vi "运维调试_五参数.vi"() -> ()   [LabVIEW 2016, in "斯坦道仪器.lvlib"]
uses:
  <vilib>/Utility/miscctls.llb/LVPointTypeDef.ctl
  PLC/PLC.lvlib
panel:
  in  "打开串口":bool
  in  "释放串口":bool
  in  "手动通电":bool
  out "多参数横条运行状态":T1(xcontrol)
  in  "数据区":i32(listbox)
  in  "探头选择":u16(ring)=9 items=["氨氮"=3, "水温"=9, "pH值"=10, "溶解氧"=11, "电导率"=12, "浊度"=13, "叶绿素a"=14, "藻密度"=15, "蓝绿藻"=16, "氧化还原电位"=17, "溶解氧%"=18, "盐度"=19]
  in  "测量数据区读取":bool
  in  "测量数据区":i32(listbox)
  in  "状态告警区读取":bool
  in  "状态告警区":i32(listbox)
  in  "自动校准":bool
  in  "读取KB":bool
  in  "写入KB":bool
  out "B":dbl caption="校准值B:"
  out "K":dbl caption="校准值K:"
  in  "校准区探头选择":u16(ring)=9 items=["氨氮"=3, "水温"=9, "pH值"=10, "电导率"=12, "浊度"=13, "叶绿素a"=14, "藻密度"=15, "蓝绿藻"=16, "氧化还原电位"=17, "溶解氧%"=18, "盐度"=19]
  in  "停止测量(单探)":bool
  in  "启动测量(单探)":bool
  in  "控制命令区探头选择":u16(ring)=9 items=["氨氮"=3, "水温"=9, "pH值"=10, "溶解氧"=11, "电导率"=12, "浊度"=13, "叶绿素a"=14, "藻密度"=15, "蓝绿藻"=16, "氧化还原电位"=17, "溶解氧%"=18, "盐度"=19]
  in  "同步时间":bool
  in  "初始化(清洗)":bool
  in  "停止测量(全部)":bool
  in  "启动测量(全部)":bool
  in  "关键参数区读取":bool
  in  "关键参数区":i32(listbox)
  in  "传感器参数读取":bool
  in  "传感器区":i32(listbox)
  in  "返回":bool
  in  "设置":bool
  out "运行状态":string
  out "开机状态":bool
  in  "停止":bool
  in  "手动启动":bool
  out "集成报警信息":string
  # "控制命令区"
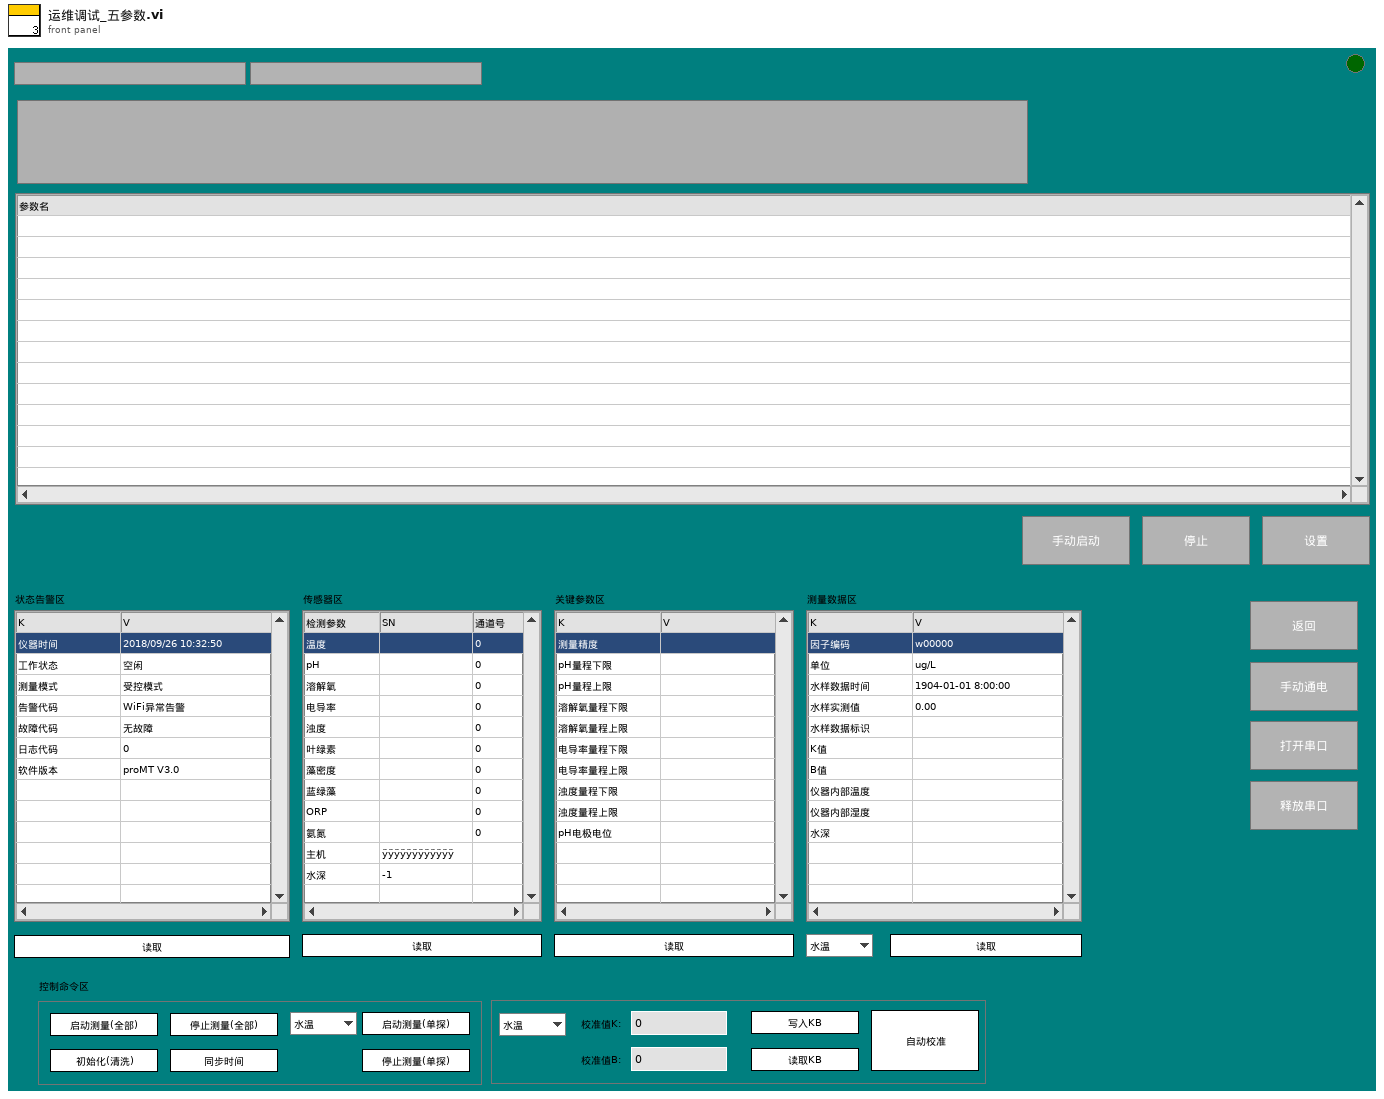
[diagram p1: front panel]
types:
  T1 = cluster{"系统时间":timestamp, "工作状态":u16, "测量模式":u16, "告警代码":enum16{"无告警", "缺试剂告警", "缺水样告警", "缺蒸馏水告警", "缺标液告警", "仪表漏液告警", "标定异常告警", "超量程告警", "加热异常", "低试剂预警", "超上限告警", "超下限告警", "仪表内部其他异常", "滴定异常告警", "电极异常告警", "量程切换告警", "参数设置告警", "PH电极电位异常", "电导率电极异常", "浊度光度异常", "溶解氧电极异常", "溶解氧光强异常", "温度异常告警", "PH异常告警", "溶解氧异常告警", "电导率异常告警", "浊度异常告警", "叶绿素异常告警", "藻密度异常告警", "蓝绿藻异常告警", "ORP异常告警", "氨氮异常告警", "清洁刷异常告警", "SD卡异常告警", "蓝牙异常告警", "Wifi异常告警", "流程异常告警"}, "故障代码":enum16{"无故障", "电机故障", "温度故障", "通讯故障", "滴定故障"}, "日志代码":u16, "软件版本":string}
  T2 = typedef "LVPointTypeDef.ctl" = cluster{"Horizontal":i16, "Vertical":i16}
  T3 = cluster{"时间标识":timestamp, "设备":string, "日志信息":string}
  T4 = enum16{"无告警", "缺试剂告警", "缺水样告警", "缺蒸馏水告警", "缺标液告警", "仪表漏液告警", "标定异常告警", "超量程告警", "加热异常", "低试剂预警", "超上限告警", "超下限告警", "仪表内部其他异常", "滴定异常告警", "电极异常告警", "量程切换告警", "参数设置告警", "PH电极电位异常", "电导率电极异常", "浊度光度异常", "溶解氧电极异常", "溶解氧光强异常", "温度异常告警", "PH异常告警", "溶解氧异常告警", "电导率异常告警", "浊度异常告警", "叶绿素异常告警", "藻密度异常告警", "蓝绿藻异常告警", "ORP异常告警", "氨氮异常告警", "清洁刷异常告警", "SD卡异常告警", "蓝牙异常告警", "Wifi异常告警", "流程异常告警"}
  T5 = cluster{"WORD[0]":u16, "WORD[1]":u16, "WORD[2]":u16, "WORD[3]":u16, "WORD[4]":u16, "WORD[5]":u16, "WORD[6]":u16, "WORD[7]":u16, "WORD[8]":u16, "WORD[9]":u16}
  T6 = cluster{"因子编码":string, "单位":string, "标样参考值":sgl, "水样数据时间":timestamp, "水样实测值":sgl, "水样数据标识":string, "K":sgl, "B":sgl, "T":sgl, "H":sgl, "水深":sgl}
  T7 = enum8{"Enabled", "Disabled", "Disabled and Grayed Out"}
  T8 = cluster{"测量模式":enum16{"待机", "水样测试", "标样核查", "零点核查", "跨度核查", "空白测试", "平行样测试", "加标回收", "空白校准", "标样校准", "初始化（清洗）"}, "数据标记表":string, "测量时间":dbl}
  T9 = cluster{"starting address":u16, "holding register value":u16}
  T10 = enum16{"idle", "init", "读状态", "读参数", "多个写入", "单个写入", "线圈写入"}
  T11 = enum32{"Bad", "Idle", "Run top level", "Running"}
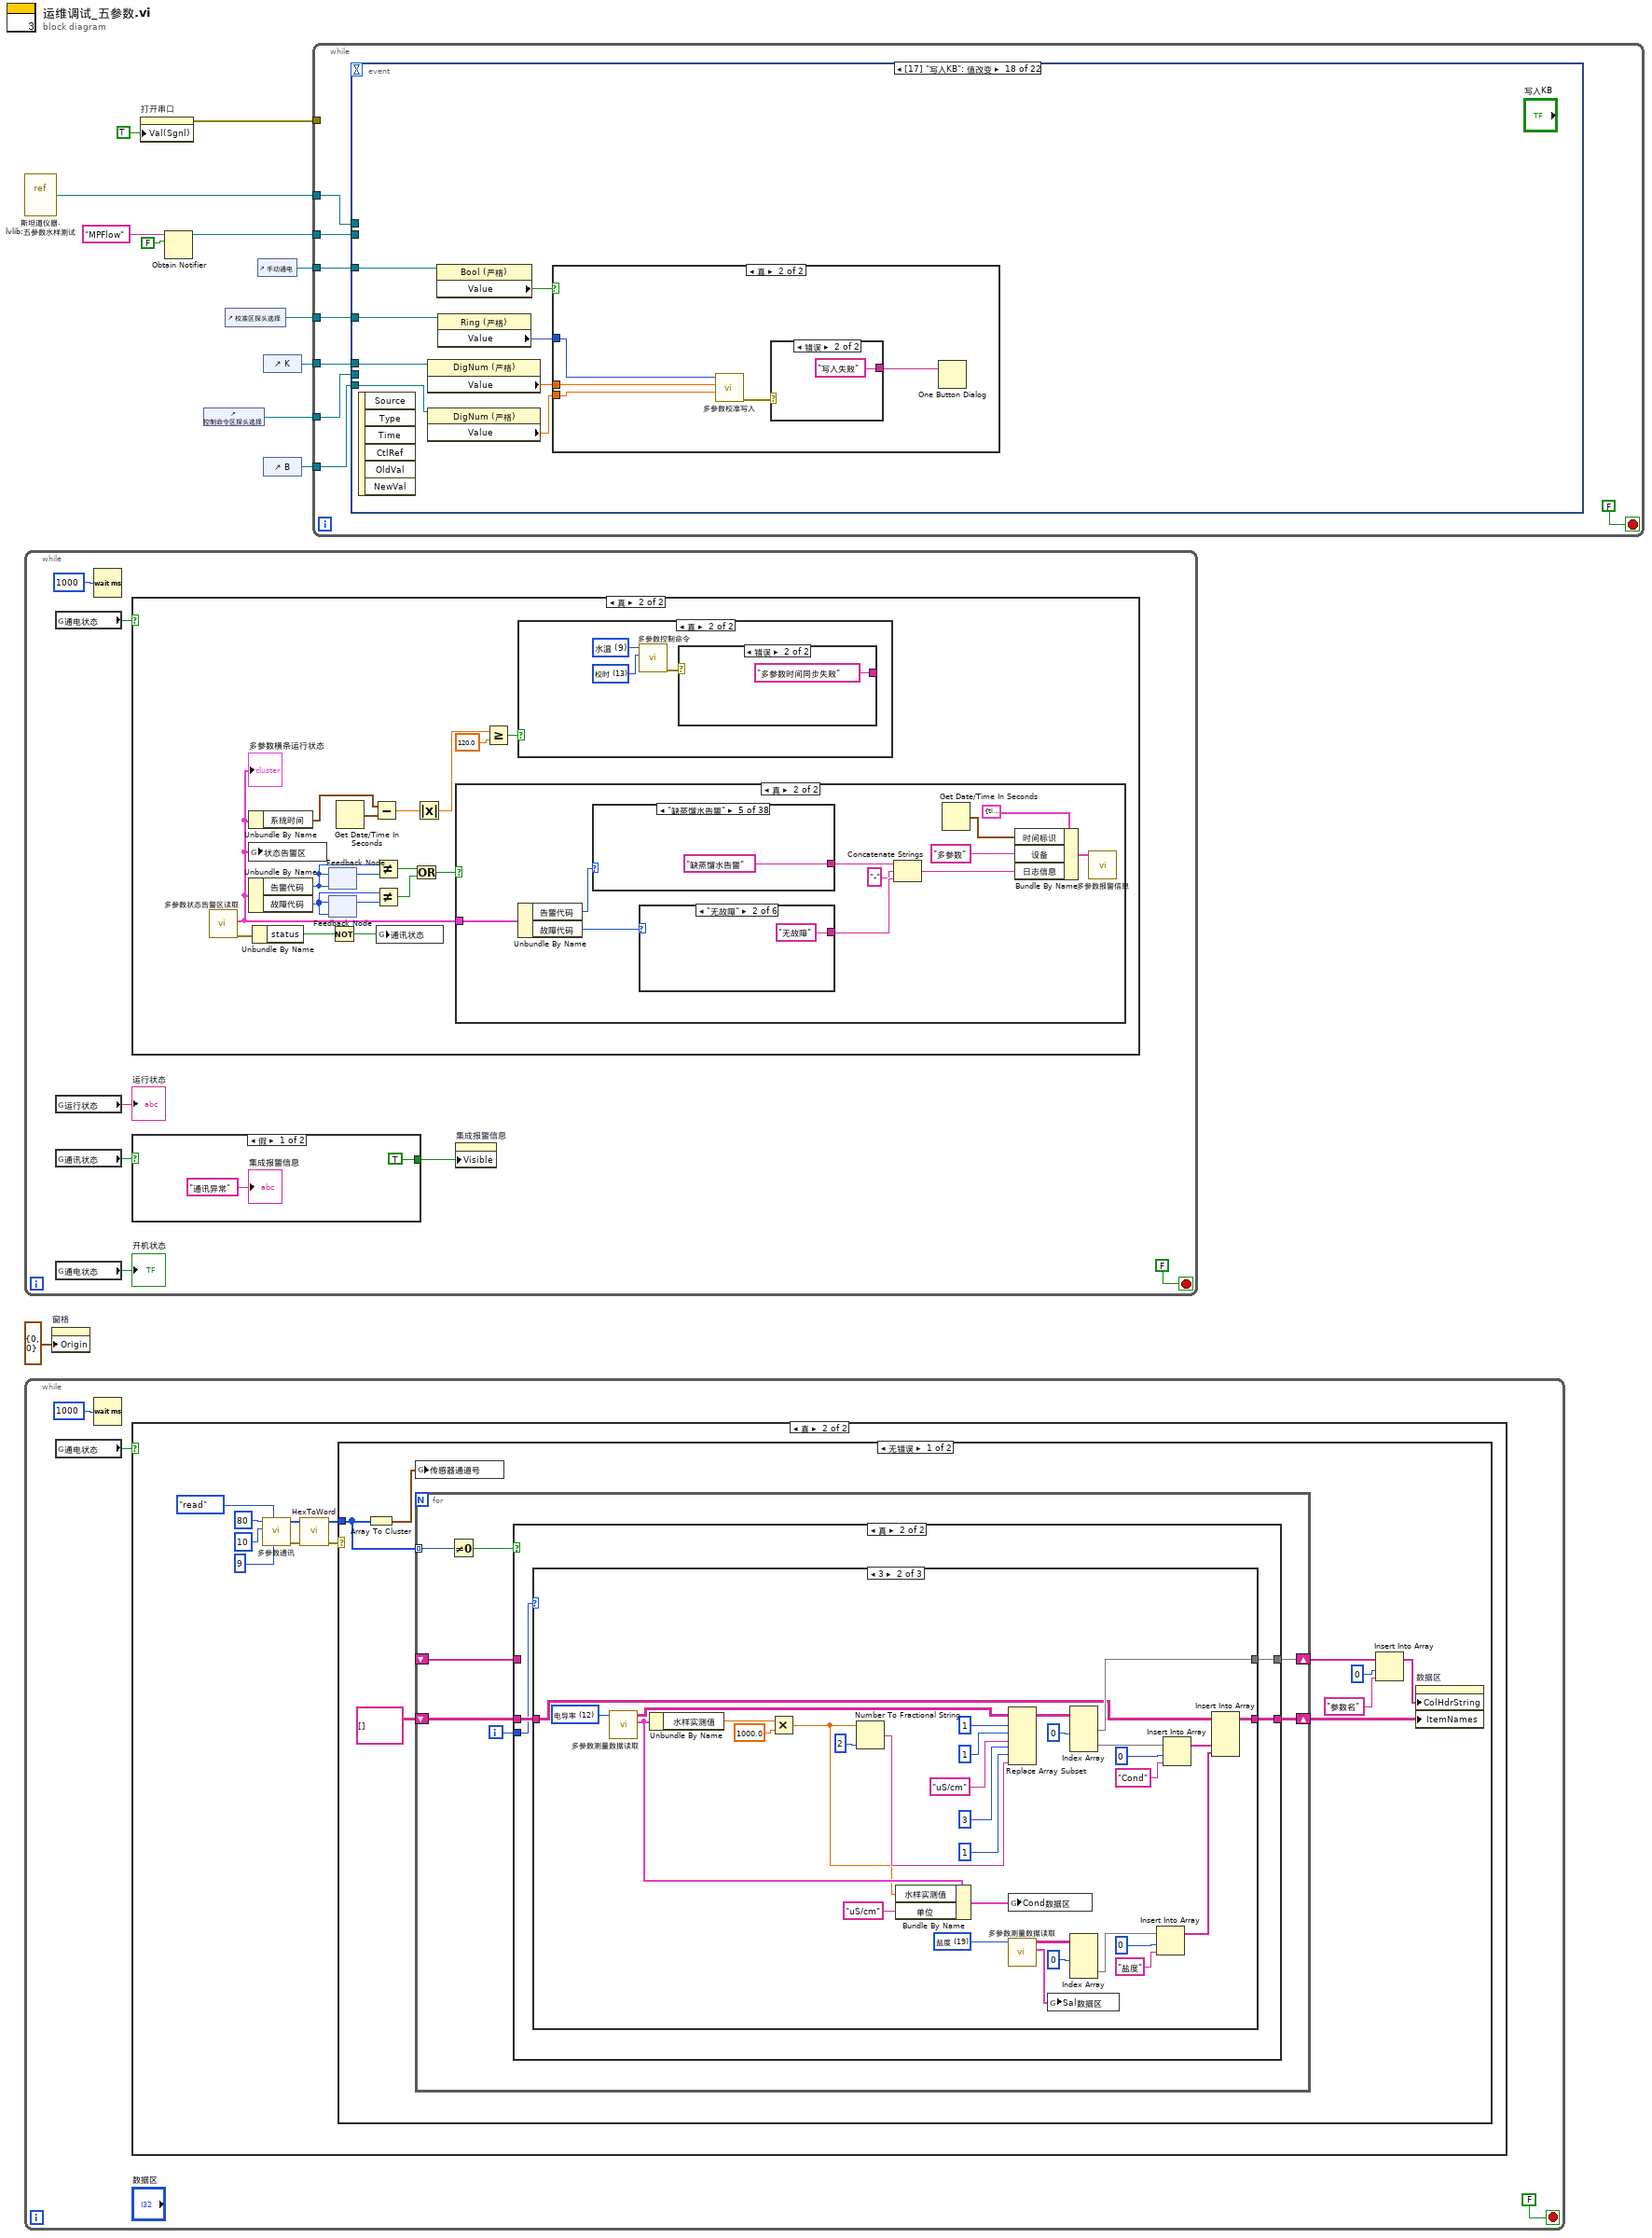
[diagram p0: block diagram]
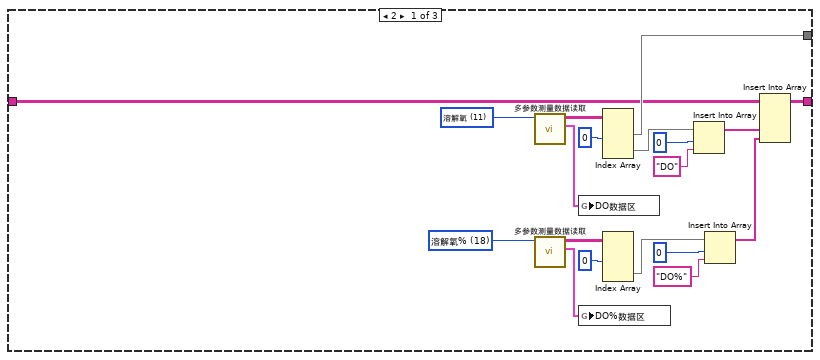
[diagram p4: hidden frame]
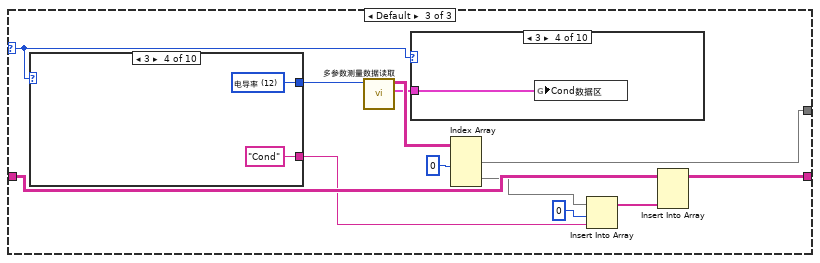
[diagram p5: hidden frame]
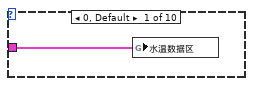
[diagram p6: hidden frame]
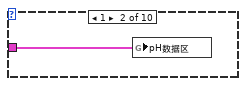
[diagram p7: hidden frame]
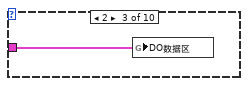
[diagram p8: hidden frame]
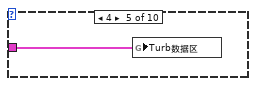
[diagram p9: hidden frame]
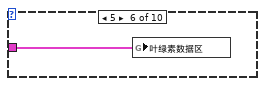
[diagram p10: hidden frame]
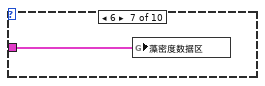
[diagram p11: hidden frame]
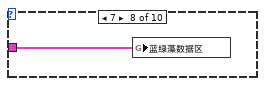
[diagram p12: hidden frame]
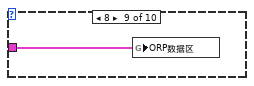
[diagram p13: hidden frame]
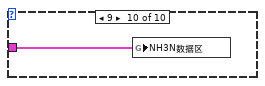
[diagram p14: hidden frame]
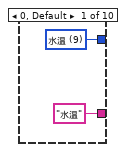
[diagram p15: hidden frame]
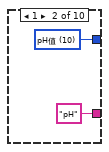
[diagram p16: hidden frame]
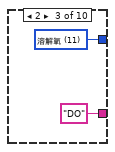
[diagram p17: hidden frame]
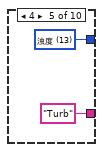
[diagram p18: hidden frame]
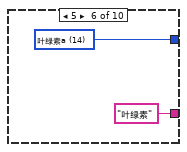
[diagram p19: hidden frame]
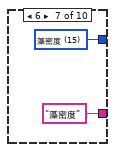
[diagram p20: hidden frame]
diagram:
  n1 = vi-ref "斯坦道仪器.lvlib:五参数水样测试.vi"() -> (w9:refnum<vi>)
  n2 = while {
    stop <- FALSE stop-if-true
    n3 = global read "多参数全局变量.vi" "通电状态"() -> (w13:bool)
    n4 = global read "多参数全局变量.vi" "运行状态"() -> (→"运行状态":string)
    n5 = global read "多参数全局变量.vi" "通讯状态"() -> (w17:bool)
    n6 = global read "多参数全局变量.vi" "通电状态"() -> (→"开机状态":bool)
    n7 = Wait (ms)(milliseconds to wait=u32 1000 ("等待时间（毫秒）")) -> ()  [unwired: 1 out]
    n8 = case shown="真" w13 {
      frame False {
      }
      frame True {
        n9 = call "多参数状态告警区读取.vi"() -> ("error out"=w29:errorcluster, "状态告警块"=w26:T1)  [unwired: 9 in, 1 out]
        "多参数横条运行状态" <- w26
        n10 = Unbundle By Name(w26) -> ("系统时间"=w25:timestamp)
        n11 = global write "多参数全局变量.vi" "状态告警区"(w26) -> ()
        n12 = Unbundle By Name(w26) -> ("告警代码"=w35:T4, "故障代码"=w33:enum16{"无故障", "电机故障", "温度故障", "通讯故障", "滴定故障"})
        n13 = Unbundle By Name(w29) -> ("status"=w28:bool)
        n14 = feedback #1(w35) -> (w36:T4)
        n15 = feedback-in #1(w35) -> ()
        n16 = feedback #2(w33) -> (w34:enum16{"无故障", "电机故障", "温度故障", "通讯故障", "滴定故障"})
        n17 = feedback-in #2(w33) -> ()
        n18 = Not(x=w28) -> (.not. x?=w27:bool)
        n19 = Get Date/Time In Seconds() -> (seconds since 1Jan1904=w24:timestamp)
        n20 = Subtract(x=w25, y=w24) -> (x-y=w23:dbl)
        n21 = Not Equal?(x=w35, y=w36) -> (x != y?=w31:bool)
        n22 = Not Equal?(x=w33, y=w34) -> (x != y?=w32:bool)
        n23 = global write "多参数全局变量.vi" "通讯状态"(w27) -> ()
        n24 = Or(x=w31, y=w32) -> (x .or. y?=w30:bool)
        n25 = Absolute Value(x=w23) -> (abs(x)=w22:dbl)
        n26 = case shown="真" w30 {
          tunnel: w26 -> [_ w52]
          frame False {
          }
          frame True {
            n27 = Unbundle By Name(w52) -> ("告警代码"=w51:T4, "故障代码"=w50:enum16{"无故障", "电机故障", "温度故障", "通讯故障", "滴定故障"})
            n28 = case shown="\"缺蒸馏水告警\"" w51 {
              selector: w51 -> [w63 _ _ _ _ _ _ _ _ _ _ _ _ _ _ _ _ _ _ _ _ _ _ _ _ _ _ _ _ _ _ _ _ _ _ _ _ _]
              tunnel: [w62 "无告警" "缺试剂告警" "缺水样告警" "缺蒸馏水告警" "缺标液告警" "仪表漏液告警" "标定异常告警" "超量程告警" "加热异常" "低试剂预警" "超上限告警" "超下限告警" "仪表内部其他异常" "滴定异常告警" "电极异常告警" "量程切换告警" "参数设置告警" "PH电极电位异常" "电导率电极异常" "浊度光度异常" "溶解氧电极异常" "溶解氧光强异常" "温度异常告警" "PH异常告警" "溶解氧异常告警" "电导率异常告警" "浊度异常告警" "叶绿素异常告警" "藻密度异常告警" "蓝绿藻异常告警" "ORP异常告警" "氨氮异常告警" "清洁刷异常告警" "SD卡异常告警" "蓝牙异常告警" "WiFi异常告警" "流程异常告警"] -> w49
              frame Default {
                n29 = Format Into String(format string="%d" ("格式字符串"), initial string="未知" ("工作状态"), w63) -> (resulting string=w62:string)  [unwired: 1 in, 1 out]
              }
              frame "无告警" {
              }
              frame "缺试剂告警" {
              }
              frame "缺水样告警" {
              }
              frame "缺蒸馏水告警" {
              }
              frame "缺标液告警" {
              }
              frame "仪表漏液告警" {
              }
              frame "标定异常告警" {
              }
              frame "超量程告警" {
              }
              frame "加热异常" {
              }
              frame "低试剂预警" {
              }
              frame "超上限告警" {
              }
              frame "超下限告警" {
              }
              frame "仪表内部其他异常" {
              }
              frame "滴定异常告警" {
              }
              frame "电极异常告警" {
              }
              frame "量程切换告警" {
              }
              frame "参数设置告警" {
              }
              frame "PH电极电位异常" {
              }
              frame "电导率电极异常" {
              }
              frame "浊度光度异常" {
              }
              frame "溶解氧电极异常" {
              }
              frame "溶解氧光强异常" {
              }
              frame "温度异常告警" {
              }
              frame "PH异常告警" {
              }
              frame "溶解氧异常告警" {
              }
              frame "电导率异常告警" {
              }
              frame "浊度异常告警" {
              }
              frame "叶绿素异常告警" {
              }
              frame "藻密度异常告警" {
              }
              frame "蓝绿藻异常告警" {
              }
              frame "ORP异常告警" {
              }
              frame "氨氮异常告警" {
              }
              frame "清洁刷异常告警" {
              }
              frame "SD卡异常告警" {
              }
              frame "蓝牙异常告警" {
              }
              frame "Wifi异常告警" {
              }
              frame "流程异常告警" {
              }
            }
            n30 = case shown="\"无故障\"" w50 {
              selector: w50 -> [w54 _ _ _ _ _]
              tunnel: [w53 "无故障" "电机故障" "温度故障" "通讯故障" "滴定故障"] -> w48
              frame Default {
                n31 = Format Into String(format string="%d" ("格式字符串"), initial string="未知" ("工作状态"), w54) -> (resulting string=w53:string)  [unwired: 1 in, 1 out]
              }
              frame "无故障" {
              }
              frame "电机故障" {
              }
              frame "温度故障" {
              }
              frame "通讯故障" {
              }
              frame "滴定故障" {
              }
            }
            n32 = Concatenate Strings(w49, "-" ("字符串"), w48) -> (w44:string)
            n33 = Get Date/Time In Seconds() -> (seconds since 1Jan1904=w43:timestamp)
            n34 = Bundle By Name(cluster=T3 {"时间标识"=timestamp(0 s since 1904-01-01), "设备"="", "日志信息"=""} ("data in"), "时间标识"=w43, "设备"="多参数", "日志信息"=w44) -> (w45:T3)
            n35 = call "多参数报警信息.vi"("data in"=w45) -> ()  [unwired: 10 in, 1 out]
          }
        }
        n36 = Greater Or Equal?(x=w22, y=120.0) -> (x >= y?=w21:bool)
        n37 = case shown="真" w21 {
          frame False {
          }
          frame True {
            w37 = u16 13 items=["启动测量（全部）"=1, "初始化（清洗）"=10, "停止测量（全部）"=11, "校时"=13, "启动测量（单个传感器）"=19, "停止测量（单个传感器）"=20] ("控制命令")
            w38 = u16 9 items=["氨氮"=3, "水温"=9, "pH值"=10, "溶解氧"=11, "电导率"=12, "浊度"=13, "叶绿素a"=14, "藻密度"=15, "蓝绿藻"=16, "氧化还原电位"=17, "溶解氧%"=18, "盐度"=19] ("站号")
            n38 = call "多参数控制命令.vi"("控制命令"=w37, "站号"=w38) -> ("error out"=w39:errorcluster)  [unwired: 9 in]
            n39 = case shown="错误" w39 {
              tunnel: ["多参数时间同步成功" ("消息") "多参数时间同步失败" ("消息")] -> _
              frame No Error {
              }
              frame Error {
              }
            }
          }
        }
      }
    }
    n40 = case shown="假" w17 {
      tunnel: [TRUE ("可见") _] -> w16
      frame False {
        "集成报警信息" <- "通讯异常" ("集成报警信息")
      }
      frame True {
      }
    }
    n41 = property on="集成报警信息" class="Str"("Visible"=w16) -> ()  [unwired: 2 in, 2 out]
  }
  n42 = while {
    stop <- FALSE stop-if-true
    n43 = global read "多参数全局变量.vi" "通电状态"() -> (w105:bool)
    n44 = Wait (ms)(milliseconds to wait=u32 1000 ("等待时间（毫秒）")) -> ()  [unwired: 1 out]
    n45 = case shown="真" w105 {
      frame False {
      }
      frame True {
        n46 = call "多参数通讯.vi"("Slave ID"=u8 9, "STEP"=enum16{"open", "read", "write", "close"}."read", "quantity"=u16 10, "starting address"=u16 80) -> ("error out"=w110:errorcluster, "Registers"=w111:u16[])  [unwired: 5 in, 1 out]
        n47 = call "HexToWord.vi"("数组"=w111) -> ("WORD"=w114:u16[])  [unwired: 10 in]
        n48 = case shown="无错误" w110 {
          tunnel: w114 -> [w115 _]
          frame No Error {
            n49 = Array To Cluster(array=w115) -> (cluster=w116:T5)
            n50 = global write "多参数全局变量.vi" "传感器通道号"(w116) -> ()
            n51 = for {
              tunnel: w115 -> [w128] mode=indexing
              shift-right: [w126] -> w120
              shift-left: _ -> [w125]
              shift-right: [w123] -> w121
              shift-left: string[][] [] ("子数组") -> [w124]
              i -> [w129]
              n52 = Not Equal To 0?(x=w128) -> (x != 0?=w127:bool)
              n53 = case shown="真" w127 {
                tunnel: w129 -> [_ w132]
                tunnel: [w131 w135] -> w126
                tunnel: w125 -> [w131 _]
                tunnel: w124 -> [w130 w134]
                tunnel: [w130 w133] -> w123
                frame False {
                }
                frame True {
                  n54 = case shown="3" w132 {
                    selector: w132 -> [_ _ w187]
                    tunnel: [w144 w176 w195] -> w135
                    tunnel: w134 -> [w140 w174 w194]
                    tunnel: [w143 w162 w193] -> w133
                    frame 2 {
                      w138 = u16 18 items=["氨氮"=3, "水温"=9, "pH值"=10, "溶解氧"=11, "电导率"=12, "浊度"=13, "叶绿素a"=14, "藻密度"=15, "蓝绿藻"=16, "氧化还原电位"=17, "溶解氧%"=18, "盐度"=19] ("探头选择")
                      w139 = u16 11 items=["氨氮"=3, "水温"=9, "pH值"=10, "溶解氧"=11, "电导率"=12, "浊度"=13, "叶绿素a"=14, "藻密度"=15, "蓝绿藻"=16, "氧化还原电位"=17, "溶解氧%"=18, "盐度"=19] ("探头选择")
                      n55 = call "多参数测量数据读取.vi"("探头选择"=w139) -> ("测量数据块"=w137:T6, "添加的数组"=w142:string[][])  [unwired: 8 in, 1 out]
                      n56 = call "多参数测量数据读取.vi"("探头选择"=w138) -> ("测量数据块"=w136:T6, "添加的数组"=w141:string[][])  [unwired: 8 in, 1 out]
                      n57 = global write "多参数全局变量.vi" "DO数据区"(w137) -> ()
                      n58 = global write "多参数全局变量.vi" "DO%数据区"(w136) -> ()
                      n59 = Index Array(array=w142, index (col) #1=0 ("禁用的索引 (列)")) -> (element #1=w144:string[], element #2=w153:string[])  [unwired: 3 in]
                      n60 = Index Array(array=w141, index (col) #1=0 ("禁用的索引 (列)")) -> (element #2=w149:string[])  [unwired: 3 in, 1 out]
                      n61 = Insert Into Array(array=w153, index=0 ("索引"), new element="DO") -> (w151:string[])
                      n62 = Insert Into Array(array=w149, index=0 ("索引"), new element="DO%") -> (w148:string[])
                      n63 = Insert Into Array(array=w140, new element #1=w151, new element #2=w148) -> (w143:string[][])  [unwired: 2 in]
                    }
                    frame 3 {
                      w172 = u16 19 items=["氨氮"=3, "水温"=9, "pH值"=10, "溶解氧"=11, "电导率"=12, "浊度"=13, "叶绿素a"=14, "藻密度"=15, "蓝绿藻"=16, "氧化还原电位"=17, "溶解氧%"=18, "盐度"=19] ("探头选择")
                      w173 = u16 12 items=["氨氮"=3, "水温"=9, "pH值"=10, "溶解氧"=11, "电导率"=12, "浊度"=13, "叶绿素a"=14, "藻密度"=15, "蓝绿藻"=16, "氧化还原电位"=17, "溶解氧%"=18, "盐度"=19] ("探头选择")
                      n64 = call "多参数测量数据读取.vi"("探头选择"=w173) -> ("测量数据块"=w168:T6, "添加的数组"=w160:string[][])  [unwired: 8 in, 1 out]
                      n65 = Unbundle By Name(w168) -> ("水样实测值"=w170:sgl)
                      n66 = Multiply(x=w170, y=sgl 1000.0) -> (x*y=w155:sgl)
                      n67 = Number To Fractional String(number=w155, precision (6)=i16 2 ("精度(6)")) -> (F-format string=w156:string)  [unwired: 2 in]
                      n68 = Bundle By Name(cluster=w168, "水样实测值"=w155, "单位"="uS/cm") -> (w166:T6)
                      n69 = Replace Array Subset(array=w160, new element #1="uS/cm" ("新元素/子数组"), index (row) #1=1 ("索引 (行)"), index (col) #1=1 ("禁用的索引 (列)"), new element #2=w156, index (row) #2=3 ("索引 (行)"), index (col) #2=1 ("禁用的索引 (列)")) -> (w161:string[][])
                      n70 = global write "多参数全局变量.vi" "Cond数据区"(w166) -> ()
                      n71 = call "多参数测量数据读取.vi"("探头选择"=w172) -> ("测量数据块"=w171:T6, "添加的数组"=w175:string[][])  [unwired: 8 in, 1 out]
                      n72 = global write "多参数全局变量.vi" "Sal数据区"(w171) -> ()
                      n73 = Index Array(array=w161, index (col) #1=0 ("禁用的索引 (列)")) -> (element #1=w176:string[], element #2=w185:string[])  [unwired: 3 in]
                      n74 = Index Array(array=w175, index (col) #1=0 ("禁用的索引 (列)")) -> (element #2=w181:string[])  [unwired: 3 in, 1 out]
                      n75 = Insert Into Array(array=w181, index=0 ("索引"), new element="盐度") -> (w180:string[])
                      n76 = Insert Into Array(array=w185, index=0 ("索引"), new element="Cond") -> (w183:string[])
                      n77 = Insert Into Array(array=w174, new element #1=w183, new element #2=w180) -> (w162:string[][])  [unwired: 2 in]
                    }
                    frame Default {
                      n78 = case shown="3" w187 {
                        tunnel: [w210 w212 w214 w216 w218 w220 w222 w224 w226 w228] -> w198
                        tunnel: ["水温" "pH" "DO" "Cond" "Turb" "叶绿素" "藻密度" "蓝绿藻" "ORP" "氨氮"] -> w191
                        frame 0, Default {
                          w210 = u16 9 items=["氨氮"=3, "水温"=9, "pH值"=10, "溶解氧"=11, "电导率"=12, "浊度"=13, "叶绿素a"=14, "藻密度"=15, "蓝绿藻"=16, "氧化还原电位"=17, "溶解氧%"=18, "盐度"=19] ("探头选择")
                        }
                        frame 1 {
                          w212 = u16 10 items=["氨氮"=3, "水温"=9, "pH值"=10, "溶解氧"=11, "电导率"=12, "浊度"=13, "叶绿素a"=14, "藻密度"=15, "蓝绿藻"=16, "氧化还原电位"=17, "溶解氧%"=18, "盐度"=19] ("探头选择")
                        }
                        frame 2 {
                          w214 = u16 11 items=["氨氮"=3, "水温"=9, "pH值"=10, "溶解氧"=11, "电导率"=12, "浊度"=13, "叶绿素a"=14, "藻密度"=15, "蓝绿藻"=16, "氧化还原电位"=17, "溶解氧%"=18, "盐度"=19] ("探头选择")
                        }
                        frame 3 {
                          w216 = u16 12 items=["氨氮"=3, "水温"=9, "pH值"=10, "溶解氧"=11, "电导率"=12, "浊度"=13, "叶绿素a"=14, "藻密度"=15, "蓝绿藻"=16, "氧化还原电位"=17, "溶解氧%"=18, "盐度"=19] ("探头选择")
                        }
                        frame 4 {
                          w218 = u16 13 items=["氨氮"=3, "水温"=9, "pH值"=10, "溶解氧"=11, "电导率"=12, "浊度"=13, "叶绿素a"=14, "藻密度"=15, "蓝绿藻"=16, "氧化还原电位"=17, "溶解氧%"=18, "盐度"=19] ("探头选择")
                        }
                        frame 5 {
                          w220 = u16 14 items=["氨氮"=3, "水温"=9, "pH值"=10, "溶解氧"=11, "电导率"=12, "浊度"=13, "叶绿素a"=14, "藻密度"=15, "蓝绿藻"=16, "氧化还原电位"=17, "溶解氧%"=18, "盐度"=19] ("探头选择")
                        }
                        frame 6 {
                          w222 = u16 15 items=["氨氮"=3, "水温"=9, "pH值"=10, "溶解氧"=11, "电导率"=12, "浊度"=13, "叶绿素a"=14, "藻密度"=15, "蓝绿藻"=16, "氧化还原电位"=17, "溶解氧%"=18, "盐度"=19] ("探头选择")
                        }
                        frame 7 {
                          w224 = u16 16 items=["氨氮"=3, "水温"=9, "pH值"=10, "溶解氧"=11, "电导率"=12, "浊度"=13, "叶绿素a"=14, "藻密度"=15, "蓝绿藻"=16, "氧化还原电位"=17, "溶解氧%"=18, "盐度"=19] ("探头选择")
                        }
                        frame 8 {
                          w226 = u16 17 items=["氨氮"=3, "水温"=9, "pH值"=10, "溶解氧"=11, "电导率"=12, "浊度"=13, "叶绿素a"=14, "藻密度"=15, "蓝绿藻"=16, "氧化还原电位"=17, "溶解氧%"=18, "盐度"=19] ("探头选择")
                        }
                        frame 9 {
                          w228 = u16 3 items=["氨氮"=3, "水温"=9, "pH值"=10, "溶解氧"=11, "电导率"=12, "浊度"=13, "叶绿素a"=14, "藻密度"=15, "蓝绿藻"=16, "氧化还原电位"=17, "溶解氧%"=18, "盐度"=19] ("探头选择")
                        }
                      }
                      n79 = call "多参数测量数据读取.vi"("探头选择"=w198) -> ("测量数据块"=w188:T6, "添加的数组"=w197:string[][])  [unwired: 8 in, 1 out]
                      n80 = case shown="3" w187 {
                        tunnel: w188 -> [w199 w200 w201 w202 w203 w204 w205 w206 w207 w208]
                        frame 0, Default {
                          n81 = global write "多参数全局变量.vi" "水温数据区"(w199) -> ()
                        }
                        frame 1 {
                          n82 = global write "多参数全局变量.vi" "pH数据区"(w200) -> ()
                        }
                        frame 2 {
                          n83 = global write "多参数全局变量.vi" "DO数据区"(w201) -> ()
                        }
                        frame 3 {
                          n84 = global write "多参数全局变量.vi" "Cond数据区"(w202) -> ()
                        }
                        frame 4 {
                          n85 = global write "多参数全局变量.vi" "Turb数据区"(w203) -> ()
                        }
                        frame 5 {
                          n86 = global write "多参数全局变量.vi" "叶绿素数据区"(w204) -> ()
                        }
                        frame 6 {
                          n87 = global write "多参数全局变量.vi" "藻密度数据区"(w205) -> ()
                        }
                        frame 7 {
                          n88 = global write "多参数全局变量.vi" "蓝绿藻数据区"(w206) -> ()
                        }
                        frame 8 {
                          n89 = global write "多参数全局变量.vi" "ORP数据区"(w207) -> ()
                        }
                        frame 9 {
                          n90 = global write "多参数全局变量.vi" "NH3N数据区"(w208) -> ()
                        }
                      }
                      n91 = Index Array(array=w197, index (col) #1=0 ("禁用的索引 (列)")) -> (element #1=w195:string[], element #2=w192:string[])  [unwired: 3 in]
                      n92 = Insert Into Array(array=w192, index=0 ("索引"), new element=w191) -> (w190:string[])
                      n93 = Insert Into Array(array=w194, new element=w190) -> (w193:string[][])  [unwired: 2 in]
                    }
                  }
                }
              }
            }
            n94 = Insert Into Array(array=w120, index=0 ("索引"), new element="参数名" ("新元素/子数组")) -> (w119:string[])
            n95 = property on="数据区" class="MCListbox (严格)"("ColHdrString"=w119, "ItemNames"=w121) -> ()  [unwired: 2 in, 2 out]
          }
          frame Error {
          }
        }
      }
    }
  }
  n96 = property on="窗格" class="Pane"("Origin"=T2 {"Horizontal"=0, "Vertical"=0} ("原点")) -> ()  [unwired: 2 in, 2 out]
  n97 = property on="打开串口" class="Bool (严格)"("Val(Sgnl)"=TRUE ("值(信号)")) -> (error out=w1:errorcluster)  [unwired: 2 in, 1 out]
  n98 = Obtain Notifier(name (unnamed)="MPFlow" ("名称（未命名）"), notification data type=FALSE) -> (notifier out=w8:refnum<notifier>)  [unwired: 2 in, 2 out]
  n99 = control-ref of="控制命令区探头选择"() -> (w7:refnum<vi>)
  n100 = control-ref of="校准区探头选择"() -> (w4:refnum<vi>)
  n101 = control-ref of="手动通电"() -> (w3:refnum<vi>)
  n102 = control-ref of="K"() -> (w6:refnum<vi>)
  n103 = control-ref of="B"() -> (w5:refnum<vi>)
  n104 = while {
    tunnel: w9 -> [w235]
    tunnel: w8 -> [w234]
    tunnel: w7 -> [w233]
    tunnel: w6 -> [w232]
    tunnel: w5 -> [w231]
    tunnel: w4 -> [w230]
    tunnel: w3 -> [w229]
    tunnel: w1 -> [_]
    stop <- FALSE stop-if-true
    n105 = event shown="[17] \"写入KB\": 值改变" {
      selector: _ -> [_ _ _ _ _ _ _ _ _ _ _ _ _ _ _ _ _ _ _ _ _ _]
      dyn-events: _ -> [_ _ _ _ _ _ _ _ _ _ _ _ _ _ _ _ _ _ _ _ _ _]
      timeout: _ -> [_ _ _ _ _ _ _ _ _ _ _ _ _ _ _ _ _ _ _ _ _ _]
      tunnel: w235 -> [_ _ _ w251 _ _ _ _ _ _ _ _ _ _ _ _ _ _ _ _ _ _]
      tunnel: w234 -> [_ _ _ _ w273 _ _ _ _ _ _ _ _ _ _ _ _ _ _ _ _ _]
      tunnel: w233 -> [_ _ _ _ _ _ _ _ _ _ _ _ _ _ _ w337 w351 _ _ _ _ _]
      tunnel: w232 -> [_ _ _ _ _ _ _ _ _ _ _ _ _ _ _ _ _ w362 _ _ _ _]
      tunnel: w231 -> [_ _ _ _ _ _ _ _ _ _ _ _ _ _ _ _ _ w364 _ _ _ _]
      tunnel: w230 -> [_ _ _ _ _ _ _ _ _ _ _ _ _ _ _ _ _ w366 _ w382 _ _]
      tunnel: w229 -> [_ _ _ _ _ _ _ w281 w286 w291 w297 w302 w311 w320 w329 w339 w349 w360 _ w380 w392 _]
      event Timeout {
        n106 = event-data() -> ()  [unwired: 1 in, 3 out]
      }
      event "释放串口": Value Change {
        n107 = event-data() -> ("NewVal"=w237:bool)  [unwired: 1 in, 5 out]
        n108 = case shown="真" w237 {
          frame False {
          }
          frame True {
            n109 = call "多参数通讯.vi"("STEP"=enum16{"open", "read", "write", "close"}."close") -> ("error out"=w238:errorcluster)  [unwired: 8 in, 2 out]
            n110 = case shown="无错误" w238 {
              frame No Error {
                n111 = property on="打开串口" class="Bool (严格)"("DisabledEnum"=T7."Enabled" ("禁用")) -> ()  [unwired: 2 in, 2 out]
              }
              frame Error {
              }
            }
          }
        }
      }
      event "打开串口": Value Change {
        n112 = event-data() -> ("NewVal"=w241:bool)  [unwired: 1 in, 5 out]
        n113 = case shown="真" w241 {
          frame False {
          }
          frame True {
            n114 = call "多参数通讯.vi"("STEP"=enum16{"open", "read", "write", "close"}."open") -> ("error out"=w242:errorcluster)  [unwired: 8 in, 2 out]
            n115 = case shown="错误" w242 {
              tunnel: [T7."Disabled and Grayed Out" ("禁用") T7."Enabled" ("禁用")] -> w244
              frame No Error {
              }
              frame Error {
                n116 = One Button Dialog(message="多参数串口打开失败" ("消息")) -> ()  [unwired: 1 in, 1 out]
              }
            }
            n117 = property on="打开串口" class="Bool (严格)"("DisabledEnum"=w244, "Value"=FALSE ("打开串口")) -> ()  [unwired: 2 in, 2 out]
          }
        }
      }
      event "手动启动": Value Change {
        n118 = event-data() -> ()  [unwired: 1 in, 6 out]
        n119 = call "多参数启动参数对话框.vi"() -> ("确认"=w250:bool, "测量时间"=w249:dbl)  [unwired: 10 in]
        n120 = case shown="真" w250 {
          tunnel: w251 -> [_ w253]
          tunnel: w249 -> [_ w252]
          frame False {
          }
          frame True {
            n121 = property class="VI"(reference=w253) -> ("Name"=w257:string, "Exec.State"=w255:T11)  [unwired: 1 in, 2 out]
            n122 = Open VI Reference(type specifier VI Refnum (for type only)=refnum<vi> refnum ("类型说明符VI引用句柄（仅用于类型）"), vi path=w257, options=128 ("选项")) -> (vi reference=w256:refnum<vi>)  [unwired: 3 in, 1 out]
            n123 = case shown="\"Idle\"" w255 {
              tunnel: w256 -> [w261 w268]
              tunnel: [w261 w267] -> w254
              tunnel: w252 -> [_ w262]
              frame "Bad", Default {
                n124 = One Button Dialog(message="仪器已经启动，无需重复启动" ("消息")) -> ()  [unwired: 1 in, 1 out]
              }
              frame "Idle" {
                n125 = global read "系统变量.vi" "运行模式"() -> (w264:enum16{"维护模式", "常规模式", "应急模式", "质控模式"})
                n126 = case shown="\"常规模式\", 默认" w264 {
                  tunnel: ["M" ("数据标记表") "hd" ("数据标记表")] -> w263
                  frame "维护模式" {
                  }
                  frame "常规模式", Default {
                  }
                }
                n127 = Bundle By Name(cluster=T8 {"测量模式"=enum."水样测试", "数据标记表"="", "测量时间"=0.0} ("启动参数"), "数据标记表"=w263, "测量时间"=w262) -> (w265:T8)
                n128 = call-by-ref "开始异步调用"(reference=w268, "启动参数"=w265) -> (reference out=w267:refnum<vi>)  [unwired: 12 in, 1 out]
              }
            }
            n129 = Close Reference(reference=w254) -> ()  [unwired: 1 in, 1 out]
          }
        }
      }
      event "停止": Value Change {
        n130 = event-data() -> ()  [unwired: 1 in, 6 out]
        n131 = Two Button Dialog(message="请再一次确认是否停止测量" ("消息")) -> (T button?=w271:bool)  [unwired: 2 in]
        n132 = case shown="真" w271 {
          tunnel: w273 -> [_ w276]
          frame False {
          }
          frame True {
            w274 = u16 11 items=["启动测量（全部）"=1, "初始化（清洗）"=10, "停止测量（全部）"=11, "校时"=13, "启动测量（单个传感器）"=19, "停止测量（单个传感器）"=20] ("控制命令")
            w275 = u16 10 items=["氨氮"=3, "水温"=9, "pH值"=10, "溶解氧"=11, "电导率"=12, "浊度"=13, "叶绿素a"=14, "藻密度"=15, "蓝绿藻"=16, "氧化还原电位"=17, "溶解氧%"=18, "盐度"=19] ("站号")
            n133 = Send Notification(notification=TRUE ("通知"), notifier=w276) -> ()  [unwired: 1 in, 2 out]
            n134 = call "多参数控制命令.vi"("控制命令"=w274, "站号"=w275) -> ()  [unwired: 9 in, 1 out]
          }
        }
      }
      event "设置": Value Change {
        n135 = event-data() -> ()  [unwired: 1 in, 6 out]
        n136 = property on="窗格" class="Pane"("Origin"=T2 {"Horizontal"=0, "Vertical"=528} ("原点")) -> ()  [unwired: 2 in, 2 out]
      }
      event "返回": Value Change {
        n137 = event-data() -> ()  [unwired: 1 in, 6 out]
        n138 = property on="窗格" class="Pane"("Origin"=T2 {"Horizontal"=0, "Vertical"=0} ("原点")) -> ()  [unwired: 2 in, 2 out]
      }
      event "传感器参数读取": Value Change {
        n139 = event-data() -> ()  [unwired: 1 in, 6 out]
        n140 = property class="Bool (严格)"(reference=w281) -> ("Value"=w280:bool)  [unwired: 1 in, 2 out]
        n141 = case shown="真" w280 {
          frame False {
            n142 = One Button Dialog(message="启动失败，请先通电" ("消息")) -> ()  [unwired: 1 in, 1 out]
          }
          frame True {
            n143 = call "多参数传感器参数读取.vi"() -> ("error out"=w283:errorcluster, "添加的数组"=w284:string[][])  [unwired: 10 in]
            n144 = call <vilib>:"General Error Handler.vi"("error in (no error)"=w283) -> ()  [unwired: 10 in, 5 out]
            n145 = property on="传感器区" class="MCListbox (严格)"("ItemNames"=w284) -> ()  [unwired: 2 in, 2 out]
          }
        }
      }
      event "关键参数区读取": Value Change {
        n146 = event-data() -> ()  [unwired: 1 in, 6 out]
        n147 = property class="Bool (严格)"(reference=w286) -> ("Value"=w285:bool)  [unwired: 1 in, 2 out]
        n148 = case shown="假" w285 {
          frame False {
            n149 = One Button Dialog(message="启动失败，请先通电" ("消息")) -> ()  [unwired: 1 in, 1 out]
          }
          frame True {
            n150 = call "多参数关键参数读取.vi"() -> ("error out"=w288:errorcluster, "添加的数组"=w289:string[][])  [unwired: 10 in]
            n151 = call <vilib>:"General Error Handler.vi"("error in (no error)"=w288) -> ()  [unwired: 10 in, 5 out]
            n152 = property on="关键参数区" class="MCListbox (严格)"("ItemNames"=w289) -> ()  [unwired: 2 in, 2 out]
          }
        }
      }
      event "测量数据区读取": Value Change {
        n153 = event-data() -> ()  [unwired: 1 in, 6 out]
        n154 = property class="Bool (严格)"(reference=w291) -> ("Value"=w290:bool)  [unwired: 1 in, 2 out]
        n155 = case shown="假" w290 {
          frame False {
            n156 = One Button Dialog(message="启动失败，请先通电" ("消息")) -> ()  [unwired: 1 in, 1 out]
          }
          frame True {
            n157 = call "多参数测量数据读取.vi"("探头选择"="探头选择") -> ("error out"=w294:errorcluster, "添加的数组"=w295:string[][])  [unwired: 8 in, 1 out]
            n158 = call <vilib>:"General Error Handler.vi"("error in (no error)"=w294) -> ()  [unwired: 10 in, 5 out]
            n159 = property on="测量数据区" class="MCListbox (严格)"("ItemNames"=w295) -> ()  [unwired: 2 in, 2 out]
          }
        }
      }
      event "状态告警区读取": Value Change {
        n160 = event-data() -> ()  [unwired: 1 in, 6 out]
        n161 = property class="Bool (严格)"(reference=w297) -> ("Value"=w296:bool)  [unwired: 1 in, 2 out]
        n162 = case shown="真" w296 {
          frame False {
            n163 = One Button Dialog(message="启动失败，请先通电" ("消息")) -> ()  [unwired: 1 in, 1 out]
          }
          frame True {
            n164 = call "多参数状态告警区读取.vi"() -> ("error out"=w299:errorcluster, "添加的数组"=w300:string[][])  [unwired: 9 in, 1 out]
            n165 = call <vilib>:"General Error Handler.vi"("error in (no error)"=w299) -> ()  [unwired: 10 in, 5 out]
            n166 = property on="状态告警区" class="MCListbox (严格)"("ItemNames"=w300) -> ()  [unwired: 2 in, 2 out]
          }
        }
      }
      event "同步时间": Value Change {
        n167 = event-data() -> ()  [unwired: 1 in, 6 out]
        n168 = property class="Bool (严格)"(reference=w302) -> ("Value"=w301:bool)  [unwired: 1 in, 2 out]
        n169 = case shown="假" w301 {
          frame False {
            n170 = One Button Dialog(message="启动失败，请先通电" ("消息")) -> ()  [unwired: 1 in, 1 out]
          }
          frame True {
            w304 = u16 13 items=["启动测量（全部）"=1, "初始化（清洗）"=10, "停止测量（全部）"=11, "校时"=13, "启动测量（单个传感器）"=19, "停止测量（单个传感器）"=20] ("控制命令")
            w305 = u16 9 items=["氨氮"=3, "水温"=9, "pH值"=10, "溶解氧"=11, "电导率"=12, "浊度"=13, "叶绿素a"=14, "藻密度"=15, "蓝绿藻"=16, "氧化还原电位"=17, "溶解氧%"=18, "盐度"=19] ("站号")
            n171 = call "多参数控制命令.vi"("控制命令"=w304, "站号"=w305) -> ("error out"=w307:errorcluster)  [unwired: 9 in]
            n172 = case shown="错误" w307 {
              tunnel: ["时间同步成功" ("消息") "时间同步失败" ("消息")] -> w306
              frame No Error {
              }
              frame Error {
              }
            }
            n173 = One Button Dialog(message=w306) -> ()  [unwired: 1 in, 1 out]
          }
        }
      }
      event "启动测量(全部)": Value Change {
        n174 = event-data() -> ()  [unwired: 1 in, 6 out]
        n175 = property class="Bool (严格)"(reference=w311) -> ("Value"=w310:bool)  [unwired: 1 in, 2 out]
        n176 = case shown="假" w310 {
          frame False {
            n177 = One Button Dialog(message="启动失败，请先通电" ("消息")) -> ()  [unwired: 1 in, 1 out]
          }
          frame True {
            w313 = u16 1 items=["启动测量（全部）"=1, "初始化（清洗）"=10, "停止测量（全部）"=11, "校时"=13, "启动测量（单个传感器）"=19, "停止测量（单个传感器）"=20] ("控制命令")
            w314 = u16 9 items=["氨氮"=3, "水温"=9, "pH值"=10, "溶解氧"=11, "电导率"=12, "浊度"=13, "叶绿素a"=14, "藻密度"=15, "蓝绿藻"=16, "氧化还原电位"=17, "溶解氧%"=18, "盐度"=19] ("站号")
            n178 = call "多参数控制命令.vi"("控制命令"=w313, "站号"=w314) -> ("error out"=w316:errorcluster)  [unwired: 9 in]
            n179 = case shown="无错误" w316 {
              tunnel: ["启动成功" ("消息") "启动失败" ("消息")] -> w315
              frame No Error {
              }
              frame Error {
              }
            }
            n180 = One Button Dialog(message=w315) -> ()  [unwired: 1 in, 1 out]
          }
        }
      }
      event "停止测量(全部)": Value Change {
        n181 = event-data() -> ()  [unwired: 1 in, 6 out]
        n182 = property class="Bool (严格)"(reference=w320) -> ("Value"=w319:bool)  [unwired: 1 in, 2 out]
        n183 = case shown="真" w319 {
          frame False {
            n184 = One Button Dialog(message="启动失败，请先通电" ("消息")) -> ()  [unwired: 1 in, 1 out]
          }
          frame True {
            w324 = u16 11 items=["启动测量（全部）"=1, "初始化（清洗）"=10, "停止测量（全部）"=11, "校时"=13, "启动测量（单个传感器）"=19, "停止测量（单个传感器）"=20] ("控制命令")
            w325 = u16 9 items=["氨氮"=3, "水温"=9, "pH值"=10, "溶解氧"=11, "电导率"=12, "浊度"=13, "叶绿素a"=14, "藻密度"=15, "蓝绿藻"=16, "氧化还原电位"=17, "溶解氧%"=18, "盐度"=19] ("站号")
            n185 = call "多参数控制命令.vi"("控制命令"=w324, "站号"=w325) -> ("error out"=w323:errorcluster)  [unwired: 9 in]
            n186 = case shown="错误" w323 {
              tunnel: ["停止成功" ("消息") "停止失败" ("消息")] -> w322
              frame No Error {
              }
              frame Error {
              }
            }
            n187 = One Button Dialog(message=w322) -> ()  [unwired: 1 in, 1 out]
          }
        }
      }
      event "初始化(清洗)": Value Change {
        n188 = event-data() -> ()  [unwired: 1 in, 6 out]
        n189 = property class="Bool (严格)"(reference=w329) -> ("Value"=w328:bool)  [unwired: 1 in, 2 out]
        n190 = case shown="真" w328 {
          frame False {
            n191 = One Button Dialog(message="启动失败，请先通电" ("消息")) -> ()  [unwired: 1 in, 1 out]
          }
          frame True {
            w333 = u16 10 items=["启动测量（全部）"=1, "初始化（清洗）"=10, "停止测量（全部）"=11, "校时"=13, "启动测量（单个传感器）"=19, "停止测量（单个传感器）"=20] ("控制命令")
            w334 = u16 9 items=["氨氮"=3, "水温"=9, "pH值"=10, "溶解氧"=11, "电导率"=12, "浊度"=13, "叶绿素a"=14, "藻密度"=15, "蓝绿藻"=16, "氧化还原电位"=17, "溶解氧%"=18, "盐度"=19] ("站号")
            n192 = call "多参数控制命令.vi"("控制命令"=w333, "站号"=w334) -> ("error out"=w331:errorcluster)  [unwired: 9 in]
            n193 = case shown="错误" w331 {
              tunnel: ["初始化成功" ("消息") "初始化失败" ("消息")] -> w332
              frame No Error {
              }
              frame Error {
              }
            }
            n194 = One Button Dialog(message=w332) -> ()  [unwired: 1 in, 1 out]
          }
        }
      }
      event "启动测量(单探)": Value Change {
        n195 = event-data() -> ()  [unwired: 1 in, 6 out]
        n196 = property class="Bool (严格)"(reference=w339) -> ("Value"=w338:bool)  [unwired: 1 in, 2 out]
        n197 = property class="Ring (严格)"(reference=w337) -> ("Value"=w340:u16)  [unwired: 1 in, 2 out]
        n198 = case shown="真" w338 {
          tunnel: w340 -> [_ w342]
          frame False {
            n199 = One Button Dialog(message="启动失败，请先通电" ("消息")) -> ()  [unwired: 1 in, 1 out]
          }
          frame True {
            w343 = u16 19 items=["启动测量（全部）"=1, "初始化（清洗）"=10, "停止测量（全部）"=11, "校时"=13, "启动测量（单个传感器）"=19, "停止测量（单个传感器）"=20] ("控制命令")
            n200 = call "多参数控制命令.vi"("控制命令"=w343, "站号"=w342) -> ("error out"=w345:errorcluster)  [unwired: 9 in]
            n201 = case shown="无错误" w345 {
              tunnel: ["启动成功" ("消息") "启动失败" ("消息")] -> w344
              frame No Error {
              }
              frame Error {
              }
            }
            n202 = One Button Dialog(message=w344) -> ()  [unwired: 1 in, 1 out]
          }
        }
      }
      event "停止测量(单探)": Value Change {
        n203 = event-data() -> ()  [unwired: 1 in, 6 out]
        n204 = property class="Bool (严格)"(reference=w349) -> ("Value"=w348:bool)  [unwired: 1 in, 2 out]
        n205 = property class="Ring (严格)"(reference=w351) -> ("Value"=w350:u16)  [unwired: 1 in, 2 out]
        n206 = case shown="真" w348 {
          tunnel: w350 -> [_ w353]
          frame False {
            n207 = One Button Dialog(message="启动失败，请先通电" ("消息")) -> ()  [unwired: 1 in, 1 out]
          }
          frame True {
            w354 = u16 20 items=["启动测量（全部）"=1, "初始化（清洗）"=10, "停止测量（全部）"=11, "校时"=13, "启动测量（单个传感器）"=19, "停止测量（单个传感器）"=20] ("控制命令")
            n208 = call "多参数控制命令.vi"("控制命令"=w354, "站号"=w353) -> ("error out"=w356:errorcluster)  [unwired: 9 in]
            n209 = case shown="错误" w356 {
              tunnel: ["停止成功" ("消息") "停止失败" ("消息")] -> w355
              frame No Error {
              }
              frame Error {
              }
            }
            n210 = One Button Dialog(message=w355) -> ()  [unwired: 1 in, 1 out]
          }
        }
      }
      event "写入KB": Value Change {
        n211 = event-data() -> ()  [unwired: 1 in, 6 out]
        n212 = property class="DigNum (严格)"(reference=w362) -> ("Value"=w361:dbl)  [unwired: 1 in, 2 out]
        n213 = property class="DigNum (严格)"(reference=w364) -> ("Value"=w363:dbl)  [unwired: 1 in, 2 out]
        n214 = property class="Bool (严格)"(reference=w360) -> ("Value"=w359:bool)  [unwired: 1 in, 2 out]
        n215 = property class="Ring (严格)"(reference=w366) -> ("Value"=w365:u16)  [unwired: 1 in, 2 out]
        n216 = case shown="真" w359 {
          tunnel: w365 -> [_ w372]
          tunnel: w363 -> [_ w371]
          tunnel: w361 -> [_ w370]
          frame False {
            n217 = One Button Dialog(message="启动失败，请先通电" ("消息")) -> ()  [unwired: 1 in, 1 out]
          }
          frame True {
            n218 = call "多参数校准写入.vi"("B"=w371, "K"=w370, "站号"=w372) -> ("error out"=w368:errorcluster)  [unwired: 8 in]
            n219 = case shown="错误" w368 {
              tunnel: ["写入成功" ("消息") "写入失败" ("消息")] -> w369
              frame No Error {
              }
              frame Error {
              }
            }
            n220 = One Button Dialog(message=w369) -> ()  [unwired: 1 in, 1 out]
          }
        }
      }
      event "K", "B": Mouse Down {
        n221 = event-data() -> ("CtlRef"=w378:refnum<vi>)  [unwired: 1 in, 5 out]
        n222 = property class="DigNum (严格)"(reference=w378) -> (reference out=w377:refnum<vi>, "Value"=w376:dbl)  [unwired: 1 in, 1 out]
        n223 = call "数字键盘.vi"("OldNumber"=w376) -> ("NewNumber"=w375:sgl)
        n224 = property class="DigNum (严格)"(reference=w377, "Value"=w375) -> ()  [unwired: 1 in, 2 out]
      }
      event "读取KB": Value Change {
        n225 = event-data() -> ()  [unwired: 1 in, 6 out]
        n226 = property class="Bool (严格)"(reference=w380) -> ("Value"=w379:bool)  [unwired: 1 in, 2 out]
        n227 = property class="Ring (严格)"(reference=w382) -> ("Value"=w381:u16)  [unwired: 1 in, 2 out]
        n228 = case shown="真" w379 {
          tunnel: w381 -> [_ w386]
          frame False {
            n229 = One Button Dialog(message="启动失败，请先通电" ("消息")) -> ()  [unwired: 1 in, 1 out]
          }
          frame True {
            n230 = call "多参校准读取.vi"("站号"=w386) -> ("error out"=w384:errorcluster, "B"=→"B":dbl, "K"=→"K":dbl)  [unwired: 8 in]
            n231 = case shown="无错误" w384 {
              tunnel: ["读取成功" ("消息") "读取失败" ("消息")] -> w385
              frame No Error {
              }
              frame Error {
              }
            }
            n232 = One Button Dialog(message=w385) -> ()  [unwired: 1 in, 1 out]
          }
        }
      }
      event "自动校准": Value Change {
        n233 = event-data() -> ()  [unwired: 1 in, 6 out]
        n234 = property class="Bool (严格)"(reference=w392) -> ("Value"=w391:bool)  [unwired: 1 in, 2 out]
        n235 = case shown="真" w391 {
          frame False {
            n236 = One Button Dialog(message="启动失败，请先通电" ("消息")) -> ()  [unwired: 1 in, 1 out]
          }
          frame True {
            n237 = call "多参校准.vi"() -> ()  [unwired: 12 in]
          }
        }
      }
      event "手动通电": Value Change {
        n238 = event-data() -> ("NewVal"=w395:bool)  [unwired: 1 in, 5 out]
        n239 = Boolean To (0,1)(Boolean=w395) -> (0, 1=w394:i16)
        n240 = Bundle By Name(cluster=T9 {"starting address"=0, "holding register value"=0}, "starting address"=u16 302, "holding register value"=w394) -> (w397:T9)
        n241 = call "采配水通讯指令.vi"("数据"=w397, "命令"=T10."单个写入") -> ()  [unwired: 10 in]
      }
    }
  }
